vi "Global Rectangle Origin & Size.vi"(11 "Global Rectangle":i32[](array[numeric])) -> (0 "Size Y":i32, 1 "Size X":i32, 2 "Origin Y":i32, 3 "Origin X":i32)   [LabVIEW 2021, in "Image.lvlib"]
uses:
  Image.lvlib
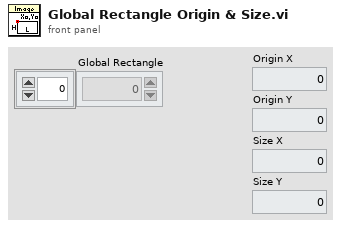
[diagram p1: front panel]
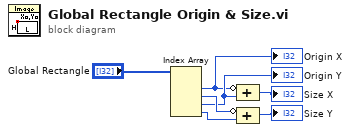
[diagram p0: block diagram]
diagram:
  n1 = Index Array(array="Global Rectangle") -> (element #1=w4:i32, element #2=w6:i32, element #3=w5:i32, element #4=w7:i32)  [unwired: 4 in]
  "Origin X" <- w4
  "Origin Y" <- w5
  n2 = Compound Arithmetic op=ADD(invert w4, w5) -> (→"Size X":i32)
  n3 = Compound Arithmetic op=ADD(invert w6, w7) -> (→"Size Y":i32)
